vi "AMC Dispatcher.vi"   [LabVIEW 2015]
doc: "This VI is used for compatibility with previous versions of the AMC library. Use the AMC VIs located in the <b>Data Communication >> Asynchronous Message Communication</b> palette."
uses:
  <vilib>/NI/AMC/AMC.lvlib
panel:
  # "Receive"
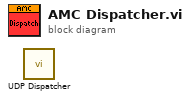
[diagram p0: block diagram]
diagram:
  n1 = call <vilib>:"UDP Dispatcher.vi"() -> ()  [unwired: 15 in, 1 out]
